vi "OCR_Test_20Jul21.vi"(0 "x":sgl=662.4014, 5 "Image File Path":path=path "C:/images/img1.jpeg", 7 "y":sgl=316.75128, 9 "Image in":T1(plugin-control), 12 "error in (no error)":errorcluster) -> (3 "Read Top":string, 6 "Read Center":string caption="Read String", 10 "Image":T1(plugin-control), 14 "Read bottom":string, 15 "error out":errorcluster)   [LabVIEW 2018]
uses:
  <vilib>/vision/NI_Vision_Development_Module.lvlib
panel:
  in  "Training File Path":path=path "D:/Focusing Station/Sub VIs/OCR_Test.abc"
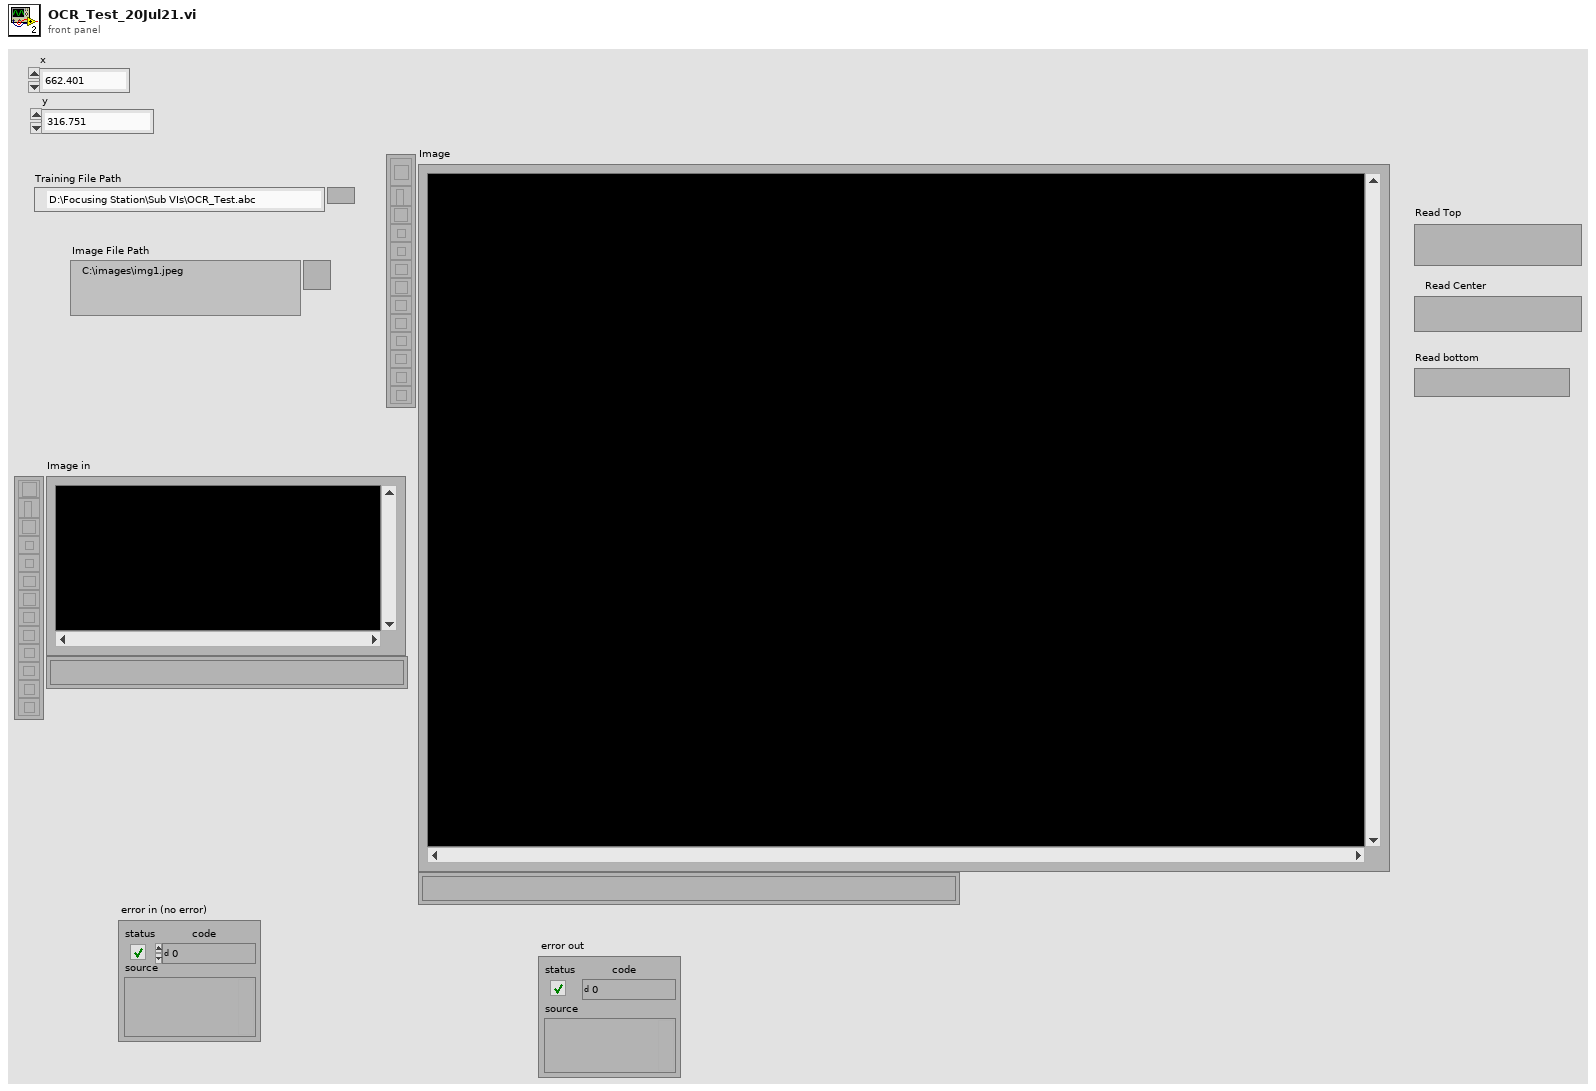
[diagram p1: front panel]
types:
  T1 = typedef "IMAQ Image.ctl" = refnum<image>
  T2 = typedef "IMAQ Rectangle" = cluster{"Left":i32, "Top":i32, "Right":i32, "Bottom":i32, "Rotation":dbl}
  T3 = typedef "Image Type" = u32
  T4 = typedef "IMAQ OCR Session.ctl" = refnum<k1>
  T5 = typedef "ROI Descriptor" = cluster{"Global Rectangle":i32[], "Contours":cluster{"ID":enum32{"External", "Internal"}, "Type":u32, "Coordinates":i32[]}[]}
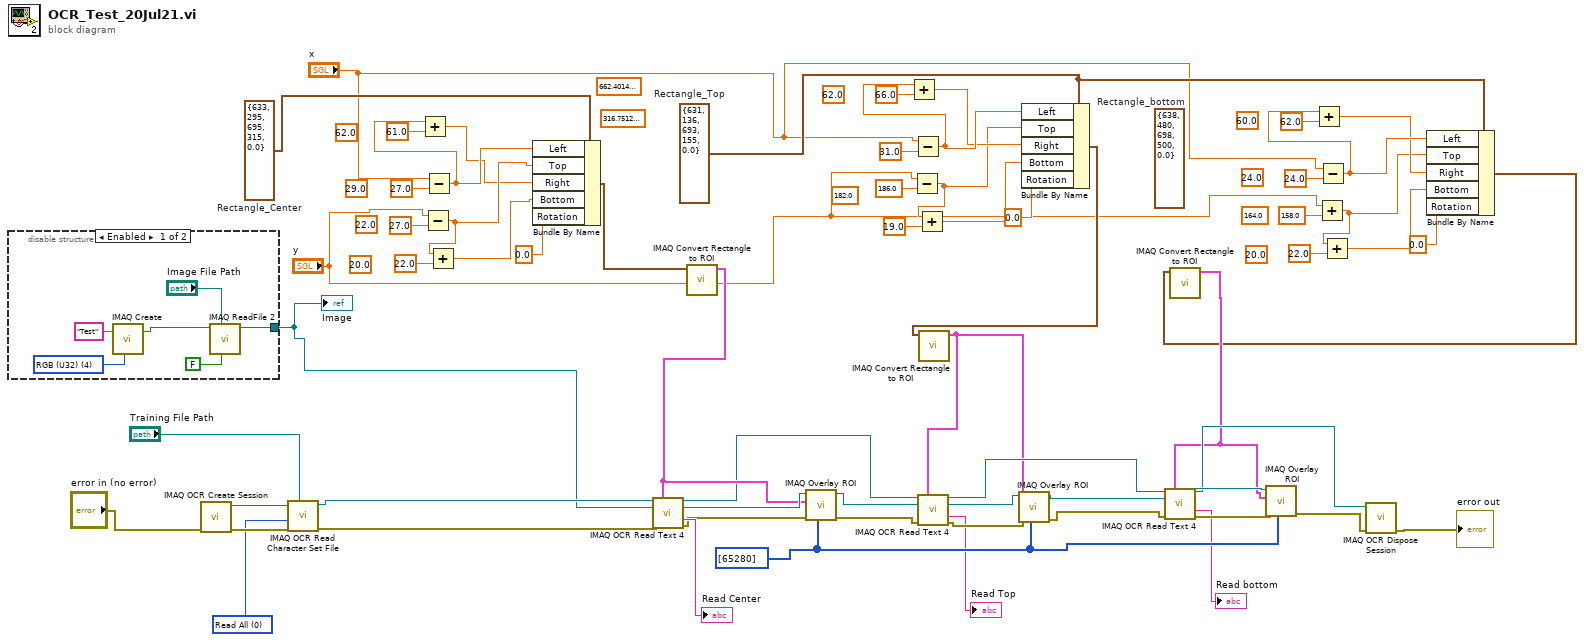
[diagram p0: block diagram]
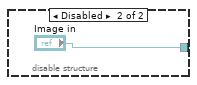
[diagram p2: hidden frame]
diagram:
  (unwired) sgl 24.0 ("y")
  (unwired) sgl 60.0 ("y")
  (unwired) sgl 20.0 ("y")
  (unwired) sgl 62.0 ("y")
  (unwired) sgl 29.0 ("y")
  (unwired) sgl 22.0 ("y")
  (unwired) sgl 20.0 ("y")
  (unwired) sgl 164.0 ("y")
  (unwired) sgl 62.0 ("y")
  (unwired) sgl 182.0 ("y")
  (unwired) sgl 316.75128 ("y")
  (unwired) sgl 662.4014 ("x")
  (unwired) T2 {"Left"=638, "Top"=480, "Right"=698, "Bottom"=500, "Rotation"=0.0}  # Rectangle_bottom
  w15 = T2 {"Left"=631, "Top"=136, "Right"=693, "Bottom"=155, "Rotation"=0.0}  # Rectangle_Top
  w55 = 0 items=["Read All", "Read Character Set Only", "Read Properties Only"] ("Read Options")
  w8 = T2 {"Left"=633, "Top"=295, "Right"=695, "Bottom"=315, "Rotation"=0.0}  # Rectangle_Center
  w39 = u32[] [65280] ("Colors (Green)")
  n1 = disable-structure shown="Enabled" {
    disable-tunnel: [w65 "Image in"] -> w59
    frame Enabled {
      w66 = T3 4 items=["Grayscale (U8)", "Grayscale (I16)", "Grayscale (SGL)", "Complex (CSG)", "RGB (U32)", "HSL (U32)", "RGB (U64)", "Grayscale (U16)"] ("Image Type")
      n2 = call "IMAQ Create"("Image Name"="Test", "Image Type"=w66) -> ("New Image"=w69:T1)  [unwired: 3 in, 1 out]
      n3 = call "IMAQ ReadFile 2"("Use File Path Image Type"=FALSE, "File Path"="Image File Path", "Image"=w69) -> ("Image Out"=w65:T1)  [unwired: 4 in, 4 out]
    }
    frame Disabled {
    }
  }
  "Image" <- w59
  n4 = call "IMAQ OCR Create Session"("error in (no error)"="error in (no error)") -> ("error out"=w63:errorcluster, "IMAQ OCR Session"=w64:T4)  [unwired: 9 in]
  n5 = call "IMAQ OCR Read Character Set File"("File Path"="Training File Path", "error in (no error)"=w63, "Read Options"=w55, "IMAQ OCR Session"=w64) -> ("error out"=w60:errorcluster, "IMAQ OCR Session (dup)"=w61:T4)  [unwired: 5 in, 1 out]
  n6 = Subtract(x="y", y=sgl 27.0) -> (x-y=w4:sgl)
  n7 = Subtract(x="x", y=sgl 27.0) -> (x-y=w5:sgl)
  n8 = Add(x=w5, y=sgl 61.0) -> (x+y=w3:sgl)
  n9 = Add(x=w4, y=sgl 22.0) -> (x+y=w2:sgl)
  n10 = Bundle By Name(cluster=w8, "Left"=w5, "Top"=w4, "Right"=w3, "Bottom"=w2, "Rotation"=0.0) -> (w1:T2)
  n11 = call "IMAQ Convert Rectangle to ROI"("Rectangle"=w1) -> ("ROI Descriptor"=w54:T5)  [unwired: 8 in, 1 out]
  n12 = call "IMAQ OCR Read Text 4"("IMAQ OCR Session"=w61, "ROI Descriptor"=w54, "Image"=w59, "error in (no error)"=w60) -> ("IMAQ OCR Session (dup)"=w49:T4, "Image (dup)"=w56:T1, "Read String"=→"Read Center":string, "error out"=w57:errorcluster)  [unwired: 5 in, 3 out]
  n13 = call "IMAQ Overlay ROI"("Colors (Green)"=w39, "error in (no error)"=w57, "ROI Descriptor"=w54, "Image"=w56) -> ("error out"=w47:errorcluster, "Image Out"=w48:T1)  [unwired: 2 in, 4 out]
  n14 = Subtract(x="y", y=sgl 186.0) -> (x-y=w27:sgl)
  n15 = Subtract(x="x", y=sgl 31.0) -> (x-y=w29:sgl)
  n16 = Add(x=w29, y=sgl 66.0) -> (x+y=w28:sgl)
  n17 = Add(x=w27, y=sgl 19.0) -> (x+y=w26:sgl)
  n18 = Bundle By Name(cluster=w15, "Left"=w29, "Top"=w27, "Right"=w28, "Bottom"=w26, "Rotation"=0.0) -> (w25:T2)
  n19 = call "IMAQ Convert Rectangle to ROI"("Rectangle"=w25) -> ("ROI Descriptor"=w35:T5)  [unwired: 8 in, 1 out]
  n20 = call "IMAQ OCR Read Text 4"("IMAQ OCR Session"=w49, "ROI Descriptor"=w35, "Image"=w48, "error in (no error)"=w47) -> ("IMAQ OCR Session (dup)"=w42:T4, "Image (dup)"=w51:T1, "Read String"=→"Read Top":string, "error out"=w50:errorcluster)  [unwired: 5 in, 3 out]
  n21 = call "IMAQ Overlay ROI"("Colors (Green)"=w39, "error in (no error)"=w50, "ROI Descriptor"=w35, "Image"=w51) -> ("error out"=w43:errorcluster, "Image Out"=w44:T1)  [unwired: 2 in, 4 out]
  n22 = Add(x="y", y=sgl 158.0) -> (x+y=w17:sgl)
  n23 = Subtract(x="x", y=sgl 24.0) -> (x-y=w19:sgl)
  n24 = Add(x=w19, y=sgl 62.0) -> (x+y=w18:sgl)
  n25 = Add(x=w17, y=sgl 22.0) -> (x+y=w16:sgl)
  n26 = Bundle By Name(cluster=w15, "Left"=w19, "Top"=w17, "Right"=w18, "Bottom"=w16, "Rotation"=0.0) -> (w14:T2)
  n27 = call "IMAQ Convert Rectangle to ROI"("Rectangle"=w14) -> ("ROI Descriptor"=w38:T5)  [unwired: 8 in, 1 out]
  n28 = call "IMAQ OCR Read Text 4"("IMAQ OCR Session"=w42, "ROI Descriptor"=w38, "Image"=w44, "error in (no error)"=w43) -> ("IMAQ OCR Session (dup)"=w41:T4, "Image (dup)"=w45:T1, "Read String"=→"Read bottom":string, "error out"=w46:errorcluster)  [unwired: 5 in, 3 out]
  n29 = call "IMAQ Overlay ROI"("Colors (Green)"=w39, "error in (no error)"=w46, "ROI Descriptor"=w38, "Image"=w45) -> ("error out"=w40:errorcluster)  [unwired: 2 in, 5 out]
  n30 = call "IMAQ OCR Dispose Session"("error in (no error)"=w40, "IMAQ OCR Session"=w41) -> ("error out"=→"error out":errorcluster)  [unwired: 9 in]
